vi "Image processing old school.vi"() -> ()   [LabVIEW 2018]
uses:
  Underlying VI's/Modified webcam FGV/Webcam AE.ctl
  <vilib>/userdefined/High Color/IMAQdx.ctl
  Underlying VI's/Elasped Timer/Elapsed timer control.ctl
  Underlying VI's/I2C Master VI/Arduino_Interfacing.ctl
  Underlying VI's/I2C Master VI/I2C_MASTER_WRITE_NEW Type Def.ctl
panel:
  out "Object detected?":bool
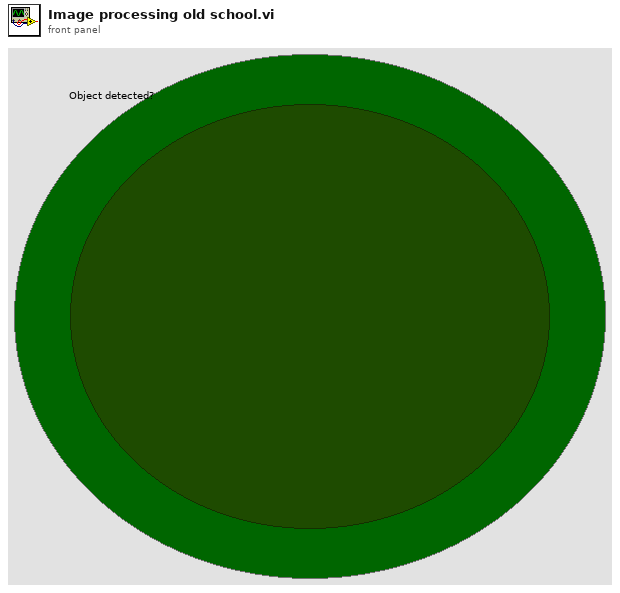
[diagram p1: front panel]
types:
  T1 = typedef "I2C_MASTER_WRITE_NEW Type Def.ctl" = enum16{"Ultrasonic sensors", "Stepper origin", "zStepper 13.3k", "zStepper 13k", "zStepper 12k", "zStepper 11k", "zStepper 10k", "zStepper 9k", "zStepper 8k", "zStepper 7k", "zStepper 6k", "zStepper 5k", "zStepper 4k", "zStepper 3k", "zStepper 2k", "zStepper 1k", "zStepper 900", "zStepper 800", "zStepper 700", "zStepper 600", "zStepper 500", "zStepper 400", "zStepper 300", "zStepper 200", "zStepper 100", "zStepper 0", "yStepper control", "Open Claw", "Close Claw", "Soft Reset"}
  T2 = typedef "Arduino_Interfacing.ctl" = enum16{"Initialize", "Write to Arduino", "Read From Arduino"}
  T3 = typedef "Webcam AE.ctl" = enum16{"Initialize Camera", "Open Camera", "Continuous Acquisition", "Close Camera", "Retrieve Image", "Dispose Camera Image Buffer"}
  T4 = typedef "Elapsed timer control.ctl" = enum16{"Start", "Pause", "Initialize"}
  T5 = typedef "IMAQdx.ctl" = refnum<k21>
  T6 = typedef "Webcam AE.ctl" = enum16{"Initialize Camera", "Open Camera", "Continuous Acquisition", "Close Camera", "Retrieve Image", "Dispose Image Buffers"}
  T7 = typedef "IMAQ Image.ctl" = refnum<image>
  T8 = cluster{"Number of Matches":i32, "Object detected?":bool}
  T9 = cluster{"Arduino State":u8, "Rotary Switch":u8, "PING A":u8, "PING B":u8, "PING C":u8, "PING D":u8, "y Stepper Position":u8, "z Stepper Position":u8, "Data Out[8]":u8}
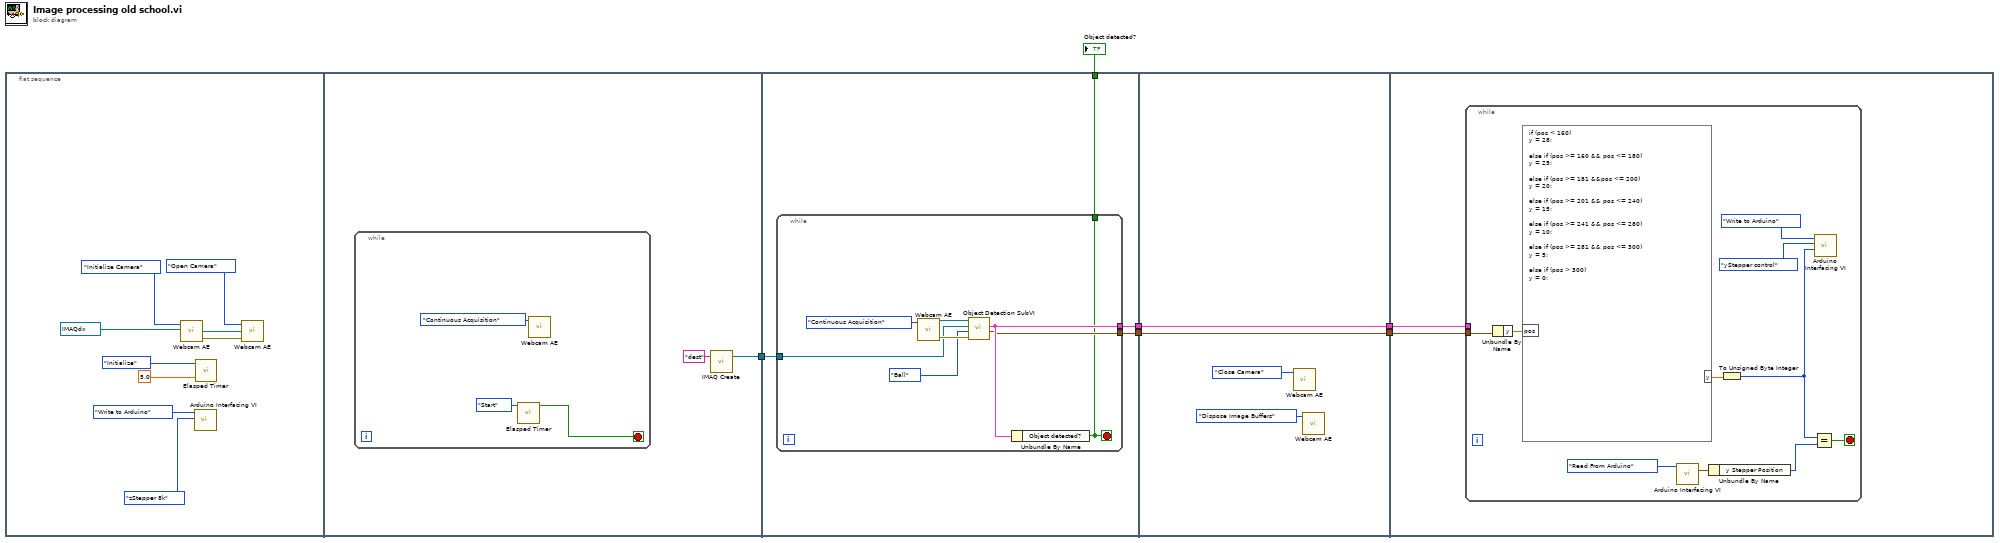
[diagram p0: block diagram]
diagram:
  n1 = flat-sequence {
    tunnel: [w16] -> w6
    tunnel: w6 -> [w24]
    tunnel: [w23] -> w5
    tunnel: [w22] -> w4
    tunnel: [w21] -> w1
    tunnel: w5 -> [w34]
    tunnel: w4 -> [w33]
    tunnel: [w34] -> w3
    tunnel: [w33] -> w2
    tunnel: w3 -> [w38]
    tunnel: w2 -> [w37]
    frame #0 {
      n2 = call "Webcam AE.vi"("Session In"=T5 "cam0", "Camera states"=Webcam_AE."Initialize Camera") -> ("error out"=w14:errorcluster, "Session Out"=w13:T5)  [unwired: 1 in, 1 out]
      n3 = call "Arduino Interfacing VI.vi"("Data to Write"=I2C_MASTER_WRITE_NEW_Type_Def."zStepper 8k", "AE Mode"=Arduino_Interfacing."Write to Arduino") -> ()  [unwired: 2 in, 2 out]
      n4 = call "Elasped Timer.vi"("Time Setting"=5.0, "Action"=Elapsed_timer_control."Initialize") -> ()  [unwired: 6 in, 4 out]
      n5 = call "Webcam AE.vi"("error in (no error)"=w14, "Session In"=w13, "Camera states"=Webcam_AE."Open Camera") -> ()  [unwired: 3 out]
    }
    frame #1 {
      n6 = while {
        stop <- w19 stop-if-true
        n7 = call "Elasped Timer.vi"("Action"=Elapsed_timer_control."Start") -> ("Time Out?!"=w19:bool)  [unwired: 7 in, 3 out]
        n8 = call "Webcam AE.vi"("Camera states"=Webcam_AE."Continuous Acquisition") -> ()  [unwired: 2 in, 3 out]
      }
      n9 = call "IMAQ Create"("Image Name"="dest") -> ("New Image"=w16:T7)  [unwired: 4 in, 1 out]
    }
    frame #2 {
      n10 = while {
        tunnel: w24 -> [w29]
        tunnel: [w27] -> w23
        tunnel: [w26] -> w22
        tunnel: [w25] -> w21
        stop <- w25 stop-if-true
        n11 = call "Webcam AE.vi"("Camera states"=Webcam_AE."Continuous Acquisition") -> ("error out"=w30:errorcluster, "Image Out"=w31:T7)  [unwired: 2 in, 1 out]
        n12 = call "Object Detection SubVI.vi"("Error In"=w30, "Mode"=enum16{"Ball", "Soap", "Gel", "Pipe", "None"}."Ball", "Image Dest"=w29, "Image in"=w31) -> ("Object Center Coordinates"=w26:cluster{"x":sgl, "y":sgl}, "Object detection cluster"=w27:T8)  [unwired: 2 out]
        n13 = Unbundle By Name(w27) -> ("Object detected?"=w25:bool)
      }
    }
    frame #3 {
      n14 = call "Webcam AE.vi"("Camera states"=Webcam_AE."Close Camera") -> ()  [unwired: 2 in, 3 out]
      n15 = call "Webcam AE.vi"("Camera states"=Webcam_AE."Dispose Image Buffers") -> ()  [unwired: 2 in, 3 out]
    }
    frame #4 {
      n16 = while {
        tunnel: w38 -> [_]
        tunnel: w37 -> [w47]
        stop <- w39 stop-if-true
        n17 = Unbundle By Name(w47) -> ("y"=w44:sgl)
        n18 = formula code="if (pos < 160)\ny = 28;\n\nelse if (pos >= 160 && pos <= 180)\ny = 25;\n\nelse if (pos >= 181 &&pos <= 200) \ny = 20;\n\nelse if (pos >= 201 && pos <= 240)\ny = 15;\n\nelse if (pos >= 241 && pos <= 280)\ny = 10;\n\nelse if (pos >= 281 && pos <= 300)\ny = 5;\n\nelse if (pos > 300)\ny = 0;"("pos"=w44) -> ("y"=w43:dbl)
        n19 = call "Arduino Interfacing VI.vi"("AE Mode"=Arduino_Interfacing."Read From Arduino") -> ("Arduino Data"=w42:T9)  [unwired: 3 in, 1 out]
        n20 = Unbundle By Name(w42) -> ("y Stepper Position"=w41:u8)
        n21 = To Unsigned Byte Integer(number=w43) -> (unsigned 8bit integer=w40:u8)
        n22 = Equal?(x=w40, y=w41) -> (x = y?=w39:bool)
        n23 = call "Arduino Interfacing VI.vi"("y Stepper value"=w40, "Data to Write"=I2C_MASTER_WRITE_NEW_Type_Def."yStepper control", "AE Mode"=Arduino_Interfacing."Write to Arduino") -> ()  [unwired: 1 in, 2 out]
      }
    }
  }
  "Object detected?" <- w1
